vi "CoordinateConvert_ArmToCartesian_Arrays.vi"(1 "ArmCoordinates":T2[](array[typedef])) -> (0 "XYPoints":T1[](array[typedef]))   [LabVIEW 2018]
uses:
  TypeDefs/ArmCoordinate.ctl
  TypeDefs/ArmAbsolutePosition.ctl
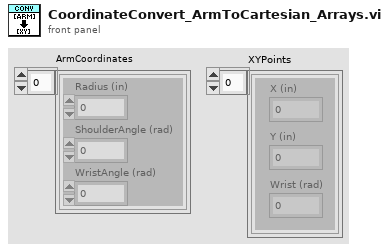
[diagram p1: front panel]
types:
  T1 = typedef "ArmAbsolutePosition.ctl" = cluster{"X (in)":dbl, "Y (in)":dbl, "Wrist (rad)":dbl}
  T2 = typedef "ArmCoordinate.ctl" = cluster{"Radius (in)":dbl, "ShoulderAngle (rad)":dbl, "WristAngle (rad)":dbl}
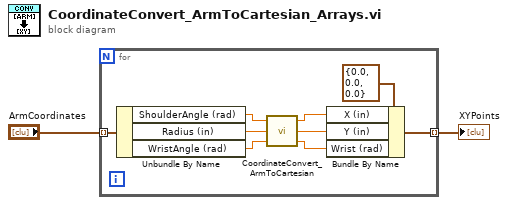
[diagram p0: block diagram]
diagram:
  n1 = for {
    tunnel: "ArmCoordinates" -> [w11] mode=indexing
    tunnel: [w5] -> w1 mode=indexing
    n2 = Unbundle By Name(w11) -> ("ShoulderAngle (rad)"=w10:dbl, "Radius (in)"=w9:dbl, "WristAngle (rad)"=w4:dbl)
    n3 = call "CoordinateConvert_ArmToCartesian.vi"("Wrist Angle (rad)"=w4, "Radius (in)"=w9, "Shoulder Angle (rad)"=w10) -> ("Wrist (rad)"=w3:dbl, "Y (in)"=w7:dbl, "X (in)"=w8:dbl)
    n4 = Bundle By Name(cluster=T1 {"X (in)"=0.0, "Y (in)"=0.0, "Wrist (rad)"=0.0} ("ArmAbsolutePose"), "X (in)"=w8, "Y (in)"=w7, "Wrist (rad)"=w3) -> (w5:T1)
  }
  "XYPoints" <- w1
